vi "WriteTriggerLog.vi"(9 "TSRefShot":bool, 10 "Trigger Data":T3, 11 "refnum In":refnum<file>) -> (3 "refnum out":refnum<file>)   [LabVIEW 2016]
uses:
  Ctrl_Signal.ctl
  Ctrl_Signal_Map.ctl
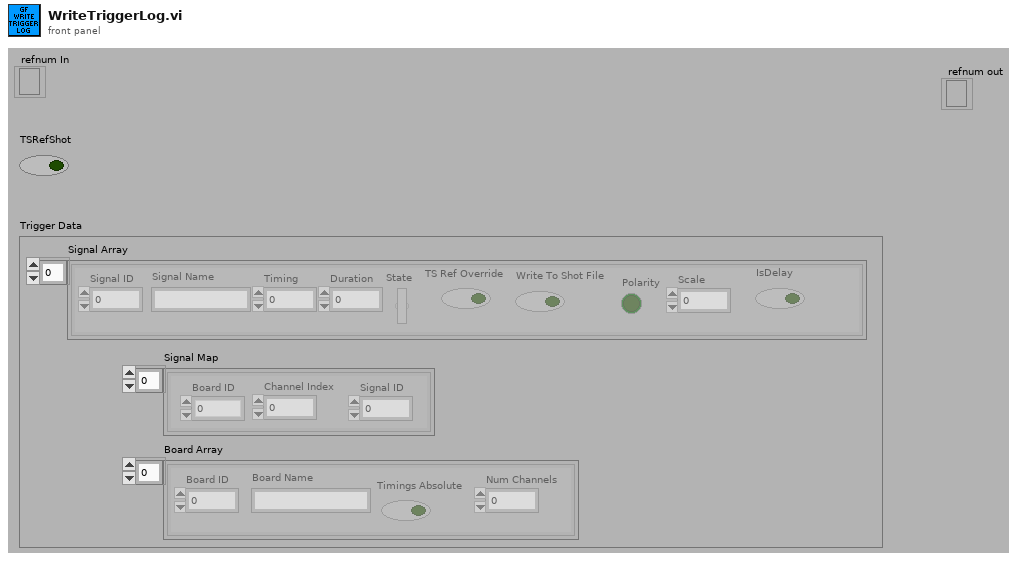
[diagram p1: front panel]
types:
  T1 = typedef "Ctrl_Signal.ctl" = cluster{"Signal Name":string, "Timing":dbl, "Duration":dbl, "State":bool, "TS Ref Override":bool, "Write To Shot File":bool, "Polarity":bool, "Signal ID":dbl, "Scale":dbl, "IsDelay":bool}
  T2 = typedef "Ctrl_Signal_Map.ctl" = cluster{"Channel Index":dbl, "Board ID":dbl, "Signal ID":dbl}
  T3 = cluster{"Signal Array":T1[], "Signal Map":T2[], "Board Array":cluster{"Board ID":dbl, "Board Name":string, "Timings Absolute":bool, "Num Channels":dbl}[]}
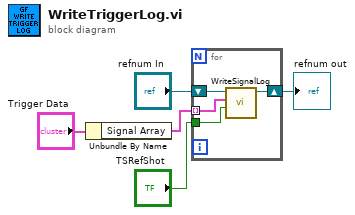
[diagram p0: block diagram]
diagram:
  n1 = Unbundle By Name("Trigger Data") -> ("Signal Array"=w4:T1[])
  n2 = for {
    tunnel: w4 -> [w9] mode=indexing
    shift-right: [w7] -> w2
    shift-left: "refnum In" -> [w8]
    tunnel: "TSRefShot" -> [w6]
    n3 = call "WriteSignalLog.vi"("TSRefShot"=w6, "Ctrl_Signal"=w9, "refnum In"=w8) -> ("refnum out"=w7:refnum<file>)  [unwired: 8 in]
  }
  "refnum out" <- w2
